vi "Constants.vi"() -> ()   [LabVIEW 2020, in "NI PXIe-4340 Shared.lvlib"]
doc: "Use this Global VI to access the GUIDs assigned to the page resources of the Custom Device."
uses:
  NI PXIe-4340 Shared.lvlib
panel:
  in  "Tab Control":enum32{"GUIDS", "Constants", "Properties"}(tab)
  in  "guids.VDT Channel":string="120e73ab-1b58-4b2a-bf69-37c104b24587"
  in  "guids.NI PXIe-4340":string="24384c3f-cbac-44b1-9e9c-67384c2c8587"
  in  "user.cd.Device.SampleRate":string="user.cd.Device.SampleRate"
  in  "user.cd.Device.DeviceName":string="user.cd.Device.DeviceName"
  in  "user.cd.Device.PhysicalChannels":string="user.cd.Device.PhysicalChannels"
  in  "user.cd.Channel.PhysicalChannel#":string="user.cd.Channel.PhysicalChannel#"
  in  "user.cd.Channel.RVDTProverties":string="user.cd.Channel.RVDTProverties"
  in  "user.cd.Channel.LVDTProperties":string="user.cd.Channel.LVDTProperties"
  in  "user.cd.Channel.InitialValue":string="user.cd.Channel.InitialValue"
  in  "user.cd.Channel.MeasurementType":string="user.cd.Channel.MeasurementType"
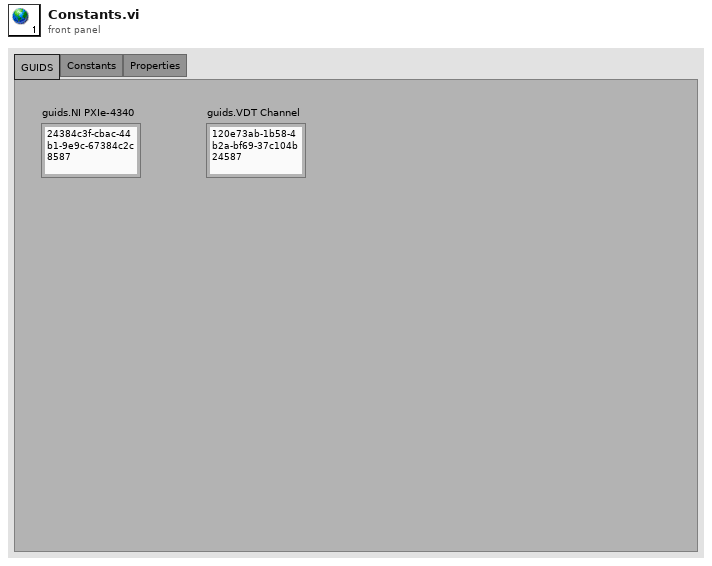
[diagram p1: front panel]
diagram:
